vi "15_HighRes.vi"(8 "error in\n(no error)":errorcluster) -> (0 "error out":errorcluster)   [LabVIEW 2014]
uses:
  SwabianInstruments.TimeTagger
panel:
  out "error message":string
  out "Mean value and RMS":dbl[][](graph)
  in  "Start TimeDifferences\nmeasurement":bool
  out "TimeDifferences data (only 40 out of 5000 bins)":i32[][](graph)
  in  "stop":bool
  in  "click_channel":i32(ring) items=["1 (Standard)"=1, "2 (Standard)"=2, "3 (Standard)"=3, "4 (Standard)"=4, "5 (Standard)"=5, "6 (Standard)"=6, "7 (Standard)"=7, "8 (Standard)"=8, "9 (Standard)"=9, "10 (Standard)"=10, "11 (Standard)"=11, "12 (Standard)"=12, "13 (Standard)"=13, "14 (Standard)"=14, "15 (Standard)"=15, "16 (Standard)"=16, "17 (Standard)"=17, "18 (Standard)"=18]
  in  "start_channel":i32(ring) items=["1 (Standard)"=1, "2 (Standard)"=2, "3 (Standard)"=3, "4 (Standard)"=4, "5 (Standard)"=5, "6 (Standard)"=6, "7 (Standard)"=7, "8 (Standard)"=8, "9 (Standard)"=9, "10 (Standard)"=10, "11 (Standard)"=11, "12 (Standard)"=12, "13 (Standard)"=13, "14 (Standard)"=14, "15 (Standard)"=15, "16 (Standard)"=16, "17 (Standard)"=17, "18 (Standard)"=18]
  in  "resolution":i32(ring) items=["Standard", "HighResA", "HighResB", "HighResC"]
  # "This example works only with a Time Tagger Ultra\nand a HighRes license.\n\n- Select a resolution -> the Time Tagger re-connects\n- Select channels to compare and start measurement\n- The Time Differences measurement will acquire 500\n   histograms, each containing 40,000 events generated\n   by the internal test signal (~50 ms per histogram)"
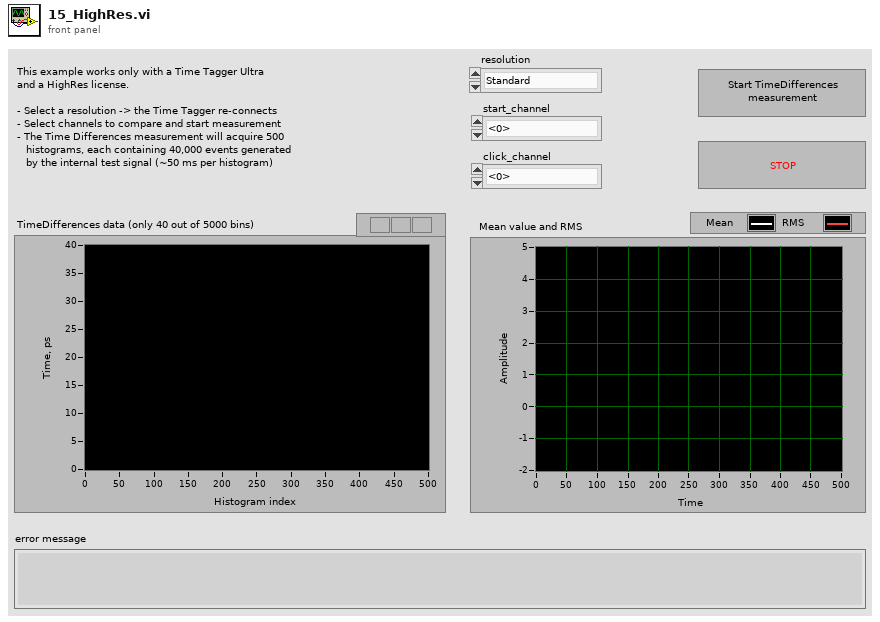
[diagram p1: front panel]
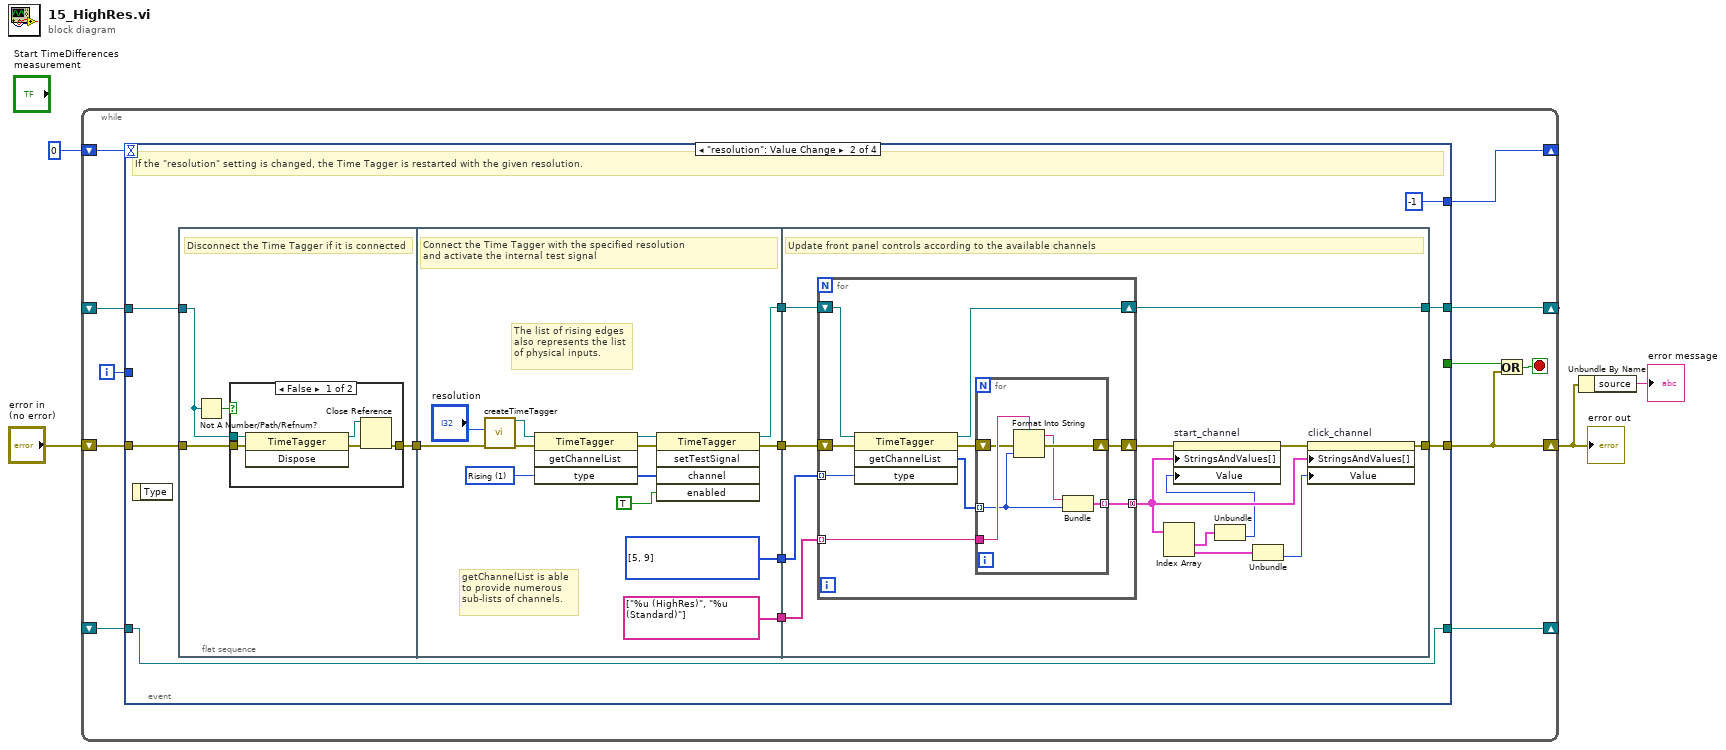
[diagram p0: block diagram]
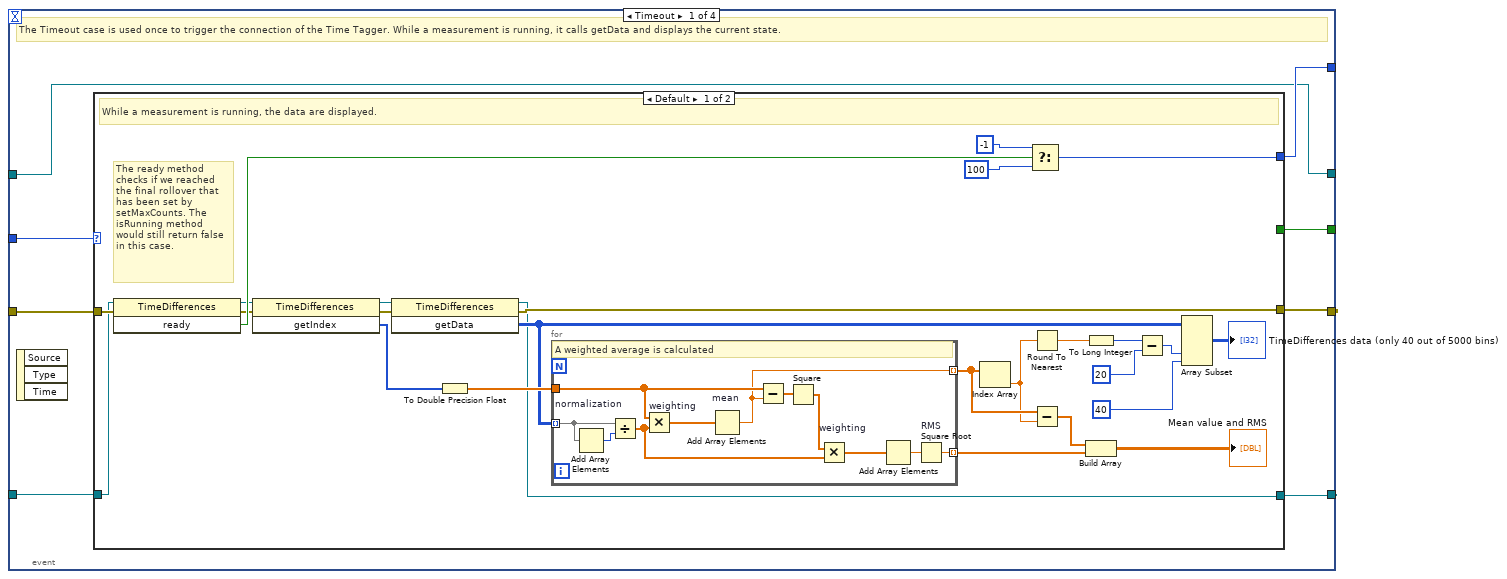
[diagram p2: hidden frame]
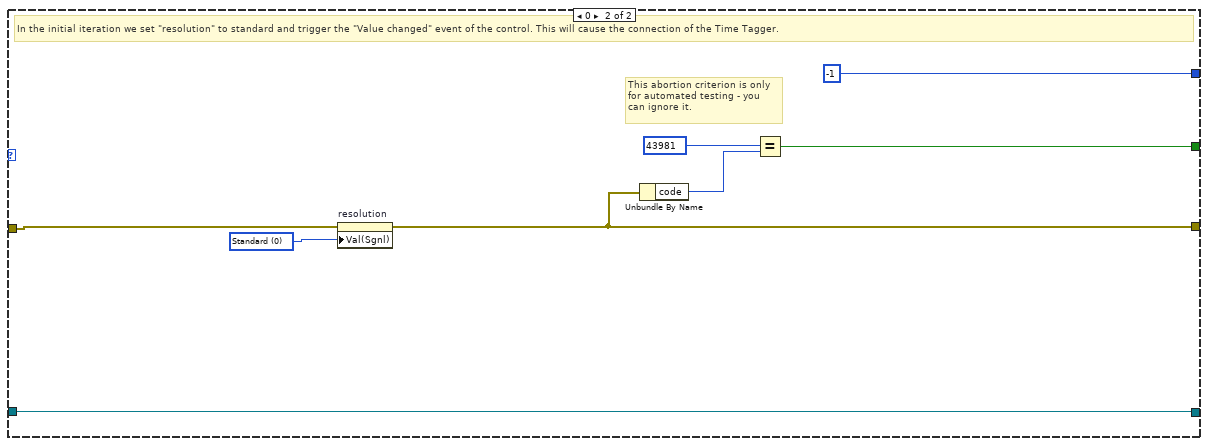
[diagram p3: hidden frame]
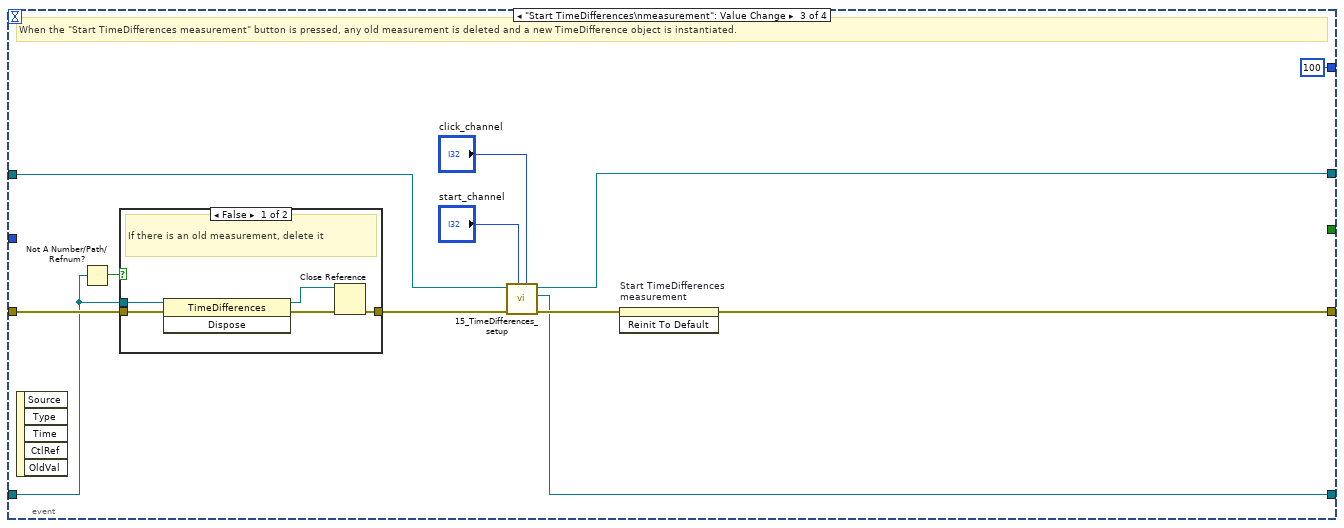
[diagram p5: hidden frame]
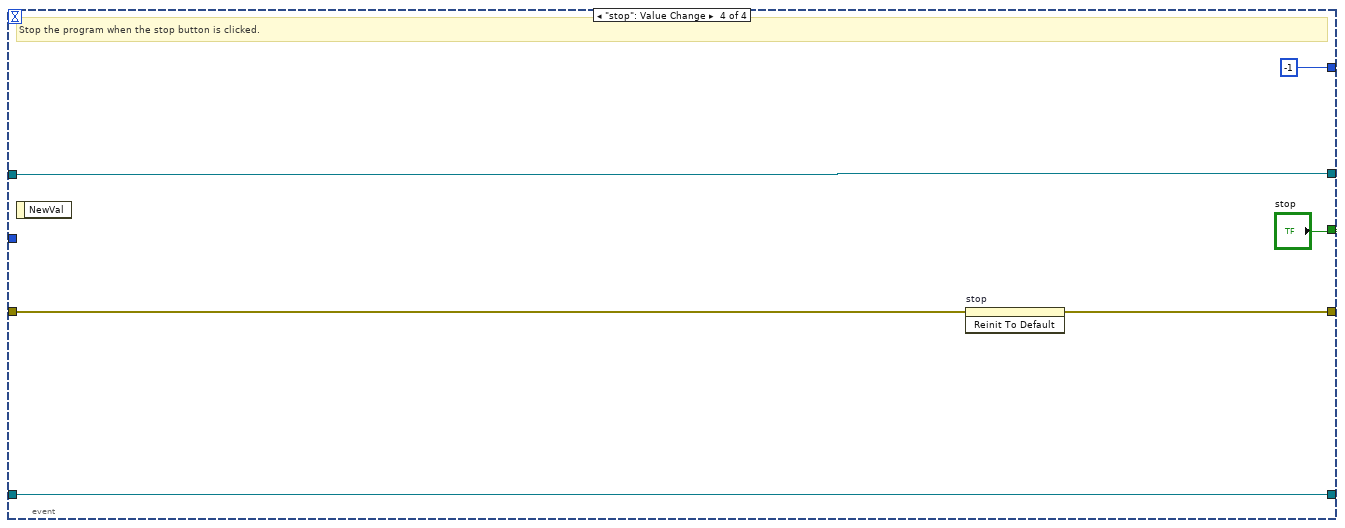
[diagram p7: hidden frame]
diagram:
  n1 = while {
    shift-right: [w15] -> _
    shift-left: _ -> [w14]
    shift-right: [w6] -> w2
    shift-left: "error in\n(no error)" -> [w13]
    shift-right: [w7] -> _
    shift-left: 0 -> [w12]
    shift-right: [w10] -> _
    shift-left: _ -> [w9]
    i -> [w11]
    stop <- w8 stop-if-true
    n2 = event shown="[1] \"resolution\": Value Change" {
      selector: _ -> [_ _ _ _]
      dyn-events: _ -> [_ _ _ _]
      timeout: w12 -> [_ _ _ _]
      tunnel: [w17 w72 w131 w153] -> w15
      tunnel: w14 -> [w17 w73 w135 w153]
      tunnel: [w16 _ _ "stop"] -> w5
      tunnel: [w21 w78 w141 w149] -> w6
      tunnel: w13 -> [w22 w75 w137 w150]
      tunnel: w11 -> [w23 _ _ _]
      tunnel: [w18 -1 100 -1 ("f")] -> w7
      tunnel: [w19 w69 w134 w154] -> w10
      tunnel: w9 -> [w20 w69 w133 w154]
      event Timeout {
        # "The Timeout case is used once to trigger the connection of the Time Tagger. While a measurement is running, it calls getData and displays the current state."
        n3 = event-data() -> ()  [unwired: 1 in, 3 out]
        n4 = case shown="Default" w23 {
          tunnel: w22 -> [w49 w67]
          tunnel: [w47 w64] -> w21
          tunnel: w20 -> [w24 w65]
          tunnel: [w44 -1] -> w18
          tunnel: [w25 w65] -> w19
          tunnel: [_ w61] -> w16
          frame Default {
            # "The ready method\nchecks if we reached\nthe final rollover that\nhas been set by\nsetMaxCounts. The\nisRunning method\nwould still return false\nin this case."
            # "While a measurement is running, the data are displayed."
            n5 = invoke class="TimeDifferences" method="ready"(reference=w24, error in=w49) -> (reference out=w43:refnum<k24>, error out=w41:errorcluster, "ready"=w48:bool)  [unwired: 1 in]
            n6 = invoke class="TimeDifferences" method="getIndex"(reference=w43, error in=w41) -> (reference out=w42:refnum<k24>, error out=w40:errorcluster, "getIndex"=w39:i64[])  [unwired: 1 in]
            n7 = invoke class="TimeDifferences" method="getData"(reference=w42, error in=w40) -> (reference out=w25:refnum<k24>, error out=w47:errorcluster, "getData"=w31:i32[][])  [unwired: 1 in]
            n8 = To Double Precision Float(number=w39) -> (double precision float=w32:dbl[])
            n9 = for {
              tunnel: w32 -> [w57]
              tunnel: w31 -> [w58] mode=indexing
              tunnel: [w56] -> w30 mode=indexing
              tunnel: [w53] -> w27 mode=indexing
              # "A weighted average is calculated"
              n10 = Add Array Elements(numeric array=w58) -> (sum=w59:i32)
              n11 = Divide "normalization"(x=w58, y=w59) -> (x/y=w55:dbl[])
              n12 = Multiply "weighting"(x=w57, y=w55) -> (x*y=w60:dbl[])
              n13 = Add Array Elements "mean"(numeric array=w60) -> (sum=w56:dbl)
              n14 = Subtract(x=w57, y=w56) -> (x-y=w52:dbl[])
              n15 = Square(x=w52) -> (x^2=w51:dbl[])
              n16 = Multiply "weighting"(x=w51, y=w55) -> (x*y=w50:dbl[])
              n17 = Add Array Elements(numeric array=w50) -> (sum=w54:dbl)
              n18 = Square Root "RMS"(x=w54) -> (sqrt(x)=w53:dbl)
            }
            n19 = Index Array(array=w30) -> (element=w29:dbl)  [unwired: 1 in]
            n20 = Select(t=-1, s=w48, f=100) -> (s? t:f=w44:i32)
            n21 = Round To Nearest(number=w29) -> (nearest integer value=w38:dbl)
            n22 = Subtract(x=w30, y=w29) -> (x-y=w28:dbl[])
            n23 = To Long Integer(number=w38) -> (32bit integer=w36:i32)
            n24 = Build Array(w28, w27) -> (→"Mean value and RMS":dbl[][])
            n25 = Subtract(x=w36, y=20) -> (x-y=w34:i32)
            n26 = Array Subset(array=w31, index (col)=w34, length (col)=40 ("length")) -> (→"TimeDifferences data (only 40 out of 5000 bins)":i32[][])  [unwired: 2 in]
          }
          frame 0 {
            w68 = 0 items=["Standard", "HighResA", "HighResB", "HighResC"] ("resolution")
            # "This abortion criterion is only\nfor automated testing - you\ncan ignore it."
            # "In the initial iteration we set \"resolution\" to standard and trigger the \"Value changed\" event of the control. This will cause the connection of the Time Tagger."
            n27 = property on="resolution" class="Ring (strict)"(error in=w67, "Val(Sgnl)"=w68) -> (error out=w64:errorcluster)  [unwired: 1 in, 1 out]
            n28 = Unbundle By Name(w64) -> ("code"=w63:i32)
            n29 = Equal?(x=43981, y=w63) -> (x = y?=w61:bool)
          }
        }
      }
      event "resolution": Value Change {
        # "If the \"resolution\" setting is changed, the Time Tagger is restarted with the given resolution."
        n30 = event-data() -> ()  [unwired: 1 in, 1 out]
        n31 = flat-sequence {
          tunnel: w75 -> [w83]
          tunnel: [w82] -> w74
          tunnel: w73 -> [w81]
          tunnel: [w96] -> w77
          tunnel: [w97] -> w76
          tunnel: w74 -> [w95]
          tunnel: [string[] ["%u (HighRes)", "%u (Standard)"]] -> w71
          tunnel: [w90] -> w70
          tunnel: [w110] -> w78
          tunnel: [w107] -> w72
          tunnel: w77 -> [w109]
          tunnel: w76 -> [w108]
          tunnel: w71 -> [w105]
          tunnel: w70 -> [w103]
          frame #0 {
            # "Disconnect the Time Tagger if it is connected"
            n32 = Not A Number/Path/Refnum?(number/path/refnum=w81) -> (NaN/Path/Refnum?=w80:bool)
            n33 = case shown="False" w80 {
              tunnel: [w88 w89] -> w82
              tunnel: w81 -> [w86 _]
              tunnel: w83 -> [w84 w89]
              frame False {
                n34 = invoke class="TimeTagger" method="Dispose"(reference=w86, error in=w84) -> (reference out=w87:refnum<k24>, error out=w85:errorcluster)  [unwired: 1 in, 1 out]
                n35 = Close Reference(reference=w87, error in (no error)=w85) -> (error out=w88:errorcluster)
              }
              frame True {
              }
            }
          }
          frame #1 {
            w90 = i32[] [5, 9] items=["All"=0, "Rising"=1, "Falling"=2, "HighResAll"=4, "HighResRising"=5, "HighResFalling"=6, "StandardAll"=8, "StandardRising"=9, "StandardFalling"=10]
            w99 = 1 items=["All"=0, "Rising"=1, "Falling"=2, "HighResAll"=4, "HighResRising"=5, "HighResFalling"=6, "StandardAll"=8, "StandardRising"=9, "StandardFalling"=10] ("type")
            # "getChannelList is able\nto provide numerous\nsub-lists of channels."
            # "The list of rising edges\nalso represents the list\nof physical inputs."
            # "Connect the Time Tagger with the specified resolution\nand activate the internal test signal"
            n36 = call "createTimeTagger.vi"("error in (no error)"=w95, "resolution"="resolution") -> ("error out"=w94:errorcluster, "TimeTagger ref out"=w92:refnum<k24>)  [unwired: 8 in]
            n37 = invoke class="TimeTagger" method="getChannelList"(reference=w92, error in=w94, "type"=w99) -> (reference out=w100:refnum<k24>, error out=w101:errorcluster, "getChannelList"=w102:i32[])  [unwired: 1 in, 1 out]
            n38 = invoke class="TimeTagger" method="setTestSignal"(reference=w100, error in=w101, "channel"=w102, "enabled"=TRUE) -> (reference out=w97:refnum<k24>, error out=w96:errorcluster)  [unwired: 1 in, 3 out]
          }
          frame #2 {
            # "Update front panel controls according to the available channels"
            n39 = for {
              tunnel: w103 -> [w124] mode=indexing
              tunnel: w105 -> [w121] mode=indexing
              tunnel: [w118] -> w106 mode=concatenating
              shift-right: [w117] -> w115
              shift-left: w109 -> [w123]
              shift-right: [w116] -> w107
              shift-left: w108 -> [w122]
              n40 = invoke class="TimeTagger" method="getChannelList"(reference=w122, error in=w123, "type"=w124) -> (reference out=w116:refnum<k24>, error out=w120:errorcluster, "getChannelList"=w119:i32[])  [unwired: 1 in, 1 out]
              n41 = for {
                tunnel: w121 -> [w130]
                tunnel: w119 -> [w128] mode=indexing
                tunnel: [w127] -> w118 mode=indexing
                shift-right: [w126] -> w117
                shift-left: w120 -> [w129]
                n42 = Format Into String(format string=w130, error in=w129, w128) -> (resulting string=w125:string, error out=w126:errorcluster)  [unwired: 1 in]
                n43 = Bundle(w125, w128) -> (w127:cluster{string, i32})  [unwired: 1 in]
              }
            }
            n44 = Index Array(array=w106) -> (element #1=w113:cluster{string, i32}, element #2=w112:cluster{string, i32})  [unwired: 2 in]
            n45 = Unbundle(w113) -> (w104:i32)  [unwired: 1 out]
            n46 = property on="start_channel" class="Ring (strict)"(error in=w115, "StringsAndValues[]"=w106, "Value"=w104) -> (error out=w114:errorcluster)  [unwired: 1 in, 1 out]
            n47 = Unbundle(w112) -> (w111:i32)  [unwired: 1 out]
            n48 = property on="click_channel" class="Ring (strict)"(error in=w114, "StringsAndValues[]"=w106, "Value"=w111) -> (error out=w110:errorcluster)  [unwired: 1 in, 1 out]
          }
        }
      }
      event "Start TimeDifferences\nmeasurement": Value Change {
        # "When the \"Start TimeDifferences measurement\" button is pressed, any old measurement is deleted and a new TimeDifference object is instantiated."
        n49 = event-data() -> ()  [unwired: 1 in, 5 out]
        n50 = Not A Number/Path/Refnum?(number/path/refnum=w133) -> (NaN/Path/Refnum?=w138:bool)
        n51 = case shown="False" w138 {
          tunnel: [w147 w148] -> w136
          tunnel: w133 -> [w145 _]
          tunnel: w137 -> [w143 w148]
          frame False {
            # "If there is an old measurement, delete it"
            n52 = invoke class="TimeDifferences" method="Dispose"(reference=w145, error in=w143) -> (reference out=w146:refnum<k24>, error out=w144:errorcluster)  [unwired: 1 in, 1 out]
            n53 = Close Reference(reference=w146, error in (no error)=w144) -> (error out=w147:errorcluster)
          }
          frame True {
          }
        }
        n54 = call "15_TimeDifferences_setup.vi"("click_channel"="click_channel", "start_channel"="start_channel", "error in (no error)"=w136, "TimeTagger ref in"=w135) -> ("error out"=w142:errorcluster, "TimeDifferences ref out"=w134:refnum<k24>, "TimeTagger ref out"=w131:refnum<k24>)  [unwired: 5 in]
        n55 = invoke on="Start TimeDifferences\nmeasurement" class="Bool" method="Reinit To Default"(error in=w142) -> (error out=w141:errorcluster)  [unwired: 2 in, 2 out]
      }
      event "stop": Value Change {
        # "Stop the program when the stop button is clicked."
        n56 = event-data() -> ()  [unwired: 1 in, 1 out]
        n57 = invoke on="stop" class="Bool" method="Reinit To Default"(error in=w150) -> (error out=w149:errorcluster)  [unwired: 2 in, 2 out]
      }
    }
    n58 = Or(x=w5, y=w6) -> (x .or. y?=w8:bool)
  }
  "error out" <- w2
  n59 = Unbundle By Name(w2) -> ("source"=→"error message":string)
